vi "GUI Panel Control.vi"(7 "action (open panel)":T1=enum."Open panel", 8 "error in (no error)":errorcluster, 11 "vi path":path) -> (0 "error out":errorcluster)   [LabVIEW 2020, in "GOLPI library.lvlib"]
doc: "Manual control of the VI panel."
uses:
  GOLPI library.lvlib
  GUI Panel Control Action.ctl
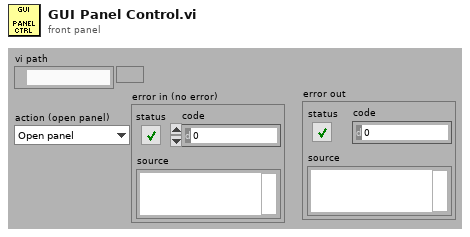
[diagram p1: front panel]
types:
  T1 = typedef "GOLPI library.lvlib/GUI Panel Control Action.ctl" = enum16{"Open hidden", "Open panel", "Close panel", "Bring To Front"}
  T2 = enum32{"Invalid", "Standard", "Closed", "Hidden", "Minimized", "Maximized"}
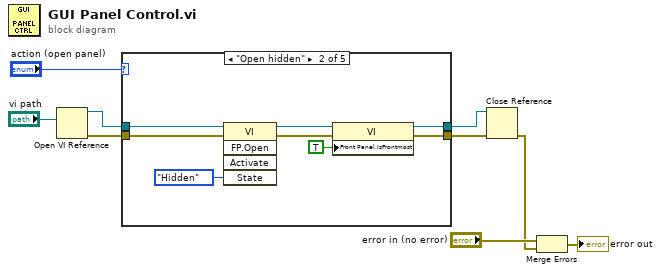
[diagram p0: block diagram]
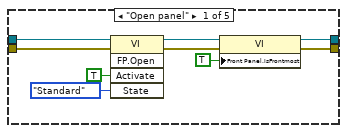
[diagram p2: hidden frame]
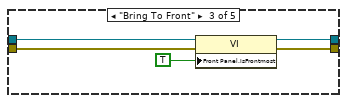
[diagram p3: hidden frame]
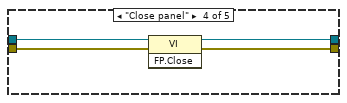
[diagram p4: hidden frame]
diagram:
  n1 = Open VI Reference(vi path="vi path") -> (vi reference=w5:refnum<vi>, error out=w7:errorcluster)  [unwired: 5 in]
  n2 = case shown="\"Open hidden\"" "action (open panel)" {
    tunnel: [w17 w25 w30 w33 w37] -> w9
    tunnel: [w16 w24 w29 w32 w36] -> w8
    tunnel: w7 -> [w15 w23 w27 w35 w37]
    tunnel: w5 -> [w14 w22 w28 w34 w36]
    frame "Open panel" {
      n3 = invoke class="VI" method="FP.Open"(reference=w14, error in=w15, "Activate"=TRUE ("Activate?"), "State"=T2."Standard") -> (reference out=w12:refnum<vi>, error out=w13:errorcluster)  [unwired: 1 in, 3 out]
      n4 = property class="VI"(reference=w12, error in=w13, "Front Panel.IsFrontmost"=TRUE ("Front Panel Window:Is Frontmost")) -> (reference out=w16:refnum<vi>, error out=w17:errorcluster)
    }
    frame "Open hidden" {
      n5 = invoke class="VI" method="FP.Open"(reference=w22, error in=w23, "State"=T2."Hidden") -> (reference out=w20:refnum<vi>, error out=w21:errorcluster)  [unwired: 2 in, 3 out]
      n6 = property class="VI"(reference=w20, error in=w21, "Front Panel.IsFrontmost"=TRUE ("Front Panel Window:Is Frontmost")) -> (reference out=w24:refnum<vi>, error out=w25:errorcluster)
    }
    frame "Bring To Front" {
      n7 = property class="VI"(reference=w28, error in=w27, "Front Panel.IsFrontmost"=TRUE ("Front Panel Window:Is Frontmost")) -> (reference out=w29:refnum<vi>, error out=w30:errorcluster)
    }
    frame "Close panel" {
      n8 = invoke class="VI" method="FP.Close"(reference=w34, error in=w35) -> (reference out=w32:refnum<vi>, error out=w33:errorcluster)  [unwired: 1 in, 1 out]
    }
    frame Default {
    }
  }
  n9 = Close Reference(reference=w8, error in (no error)=w9) -> (error out=w2:errorcluster)
  n10 = Merge Errors("error in (no error)", w2) -> (→"error out":errorcluster)
